vi "Configure Measurement.vi"(6 "Manual Range (1.00)":dbl=1.0 format="%_3f", 7 "Manual Resolution (5.5 Digits)":dbl(ring)=5.5 items=["4.5"=4.5, "5.5"=5.5, "6.5"=6.5], 8 "error in (no error)":errorcluster, 9 "Enable Auto Range (T: Enable)":bool=TRUE, 10 "Function (0: DC Voltage)":u16(ring) items=["DC Voltage", "AC Voltage", "2 - Wire Resistance", "4 - Wire Resistance", "DC Current", "AC Current", "Frequency", "Period", "Continuity", "Diode Checking", "VDC:VDC Ratio", "Temperature", "Capacitance"], 11 "VISA resource name":refnum<visa-resource-name>) -> (0 "error out":errorcluster, 3 "VISA resource name out":refnum<visa-resource-name>)   [LabVIEW 2013, in "Agilent 34401.lvlib"]
doc: "Configures the measurement type, resolution, and range on the instrument.\n\n<B>Note:</B>\n\nThis VI must be called before other configuration VIs."
uses:
  <instrlib>/Agilent 34401/Agilent 34401.lvlib
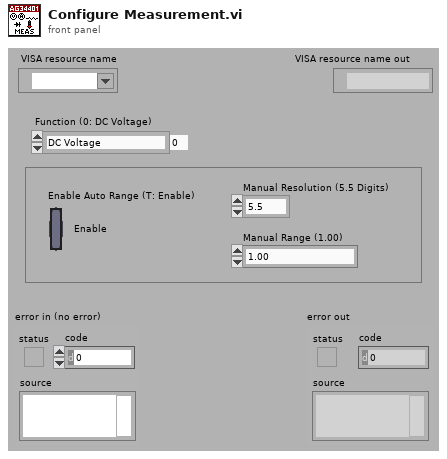
[diagram p1: front panel]
types:
  T1 = typedef "Agilent 34401.lvlib/Extended User Data.ctl" = cluster{"Trigger Source":u16, "Math Storage":u16, "Agilent Model":i32}
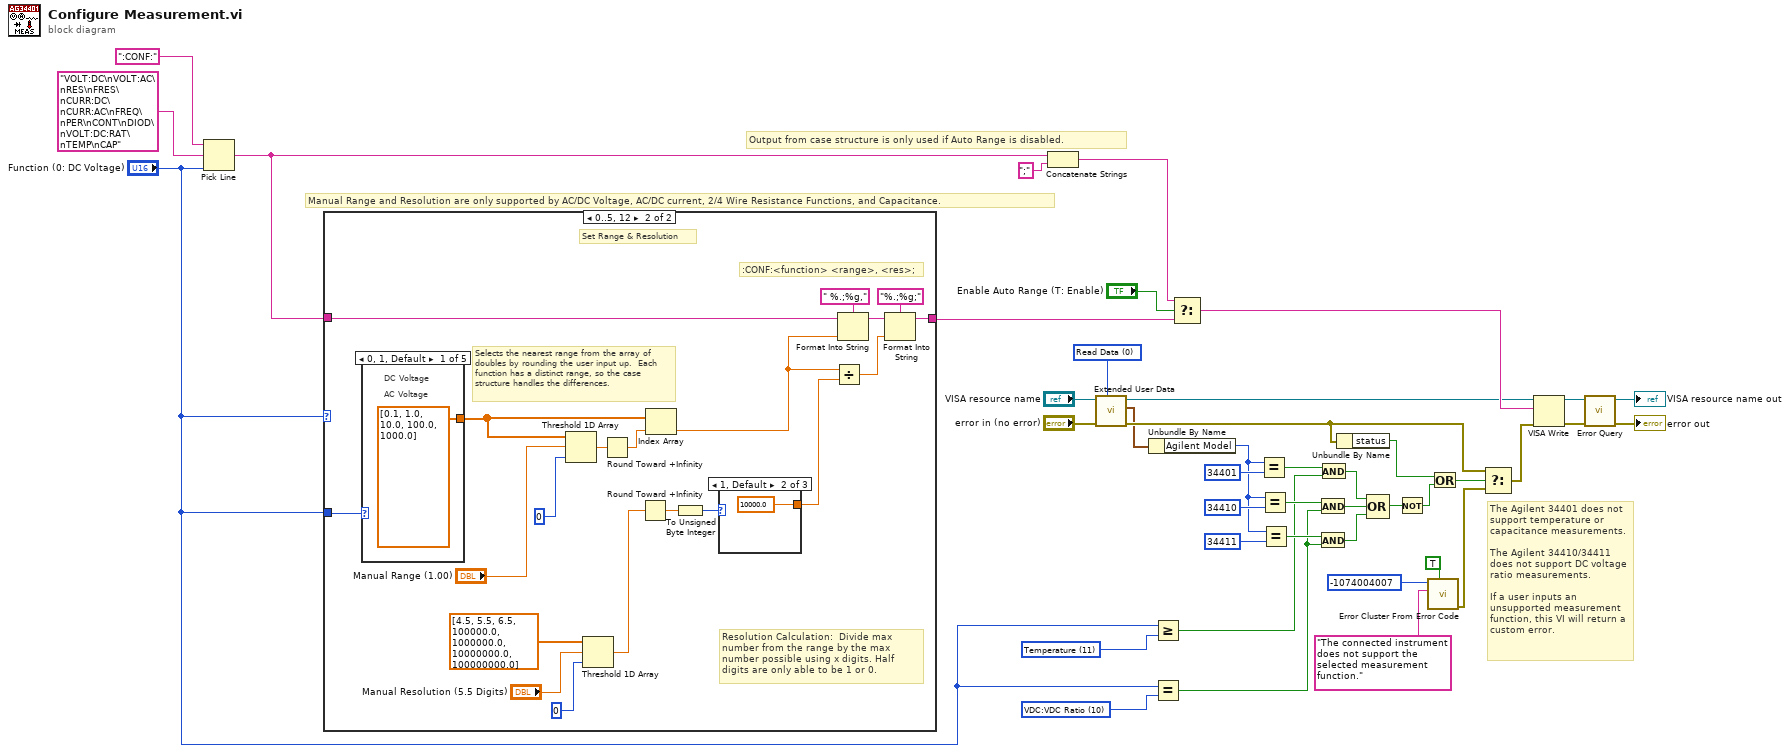
[diagram p0: block diagram]
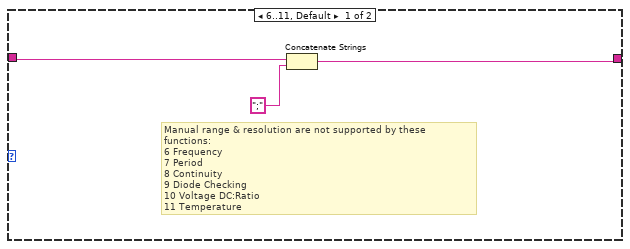
[diagram p2: hidden frame]
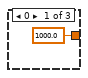
[diagram p3: hidden frame]
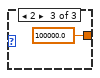
[diagram p4: hidden frame]
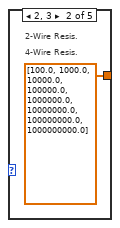
[diagram p5: hidden frame]
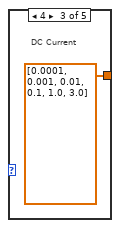
[diagram p6: hidden frame]
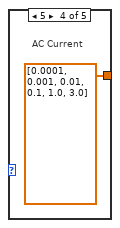
[diagram p7: hidden frame]
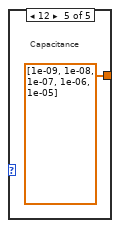
[diagram p8: hidden frame]
diagram:
  w4 = u16 10 items=["DC Voltage", "AC Voltage", "2 - Wire Resistance", "4 - Wire Resistance", "DC Current", "AC Current", "Frequency", "Period", "Continuity", "Diode Checking", "VDC:VDC Ratio", "Temperature", "Capacitance"] ("Function (0: DC Voltage)")
  w3 = u16 11 items=["DC Voltage", "AC Voltage", "2 - Wire Resistance", "4 - Wire Resistance", "DC Current", "AC Current", "Frequency", "Period", "Continuity", "Diode Checking", "VDC:VDC Ratio", "Temperature", "Capacitance"] ("Function (0: DC Voltage)")
  w6 = u16 0 items=["Read Data", "Write Data", "Dispose of Data"] ("Action")
  # "The Agilent 34401 does not support temperature or capacitance measurements.\n\nThe Agilent 34410/34411 does not support DC voltage ratio measurements.\n\nIf a user inputs an unsupported measurement function, this VI will return a custom error."
  # "Manual Range and Resolution are only supported by AC/DC Voltage, AC/DC current, 2/4 Wire Resistance Functions, and Capacitance."
  # "Output from case structure is only used if Auto Range is disabled."
  n1 = Pick Line(string ("")=":CONF:", multi-line string="VOLT:DC\nVOLT:AC\nRES\nFRES\nCURR:DC\nCURR:AC\nFREQ\nPER\nCONT\nDIOD\nVOLT:DC:RAT\nTEMP\nCAP", line index="Function (0: DC Voltage)") -> (output string=w31:string)
  n2 = case shown="0..5, 12" "Function (0: DC Voltage)" {
    tunnel: w31 -> [w45 w46]
    tunnel: "Function (0: DC Voltage)" -> [_ w56]
    tunnel: [w43 w54] -> w36
    frame 6..11, Default {
      # "Manual range & resolution are not supported by these functions:\n6 Frequency\n7 Period\n8 Continuity\n9 Diode Checking\n10 Voltage DC:Ratio\n11 Temperature"
      n3 = Concatenate Strings(w45, ";" ("Auto Range")) -> (w43:string)
    }
    frame 0..5, 12 {
      # "Set Range & Resolution"
      # ":CONF:<function> <range>, <res>;"
      # "Resolution Calculation:  Divide max number from the range by the max number possible using x digits. Half digits are only able to be 1 or 0."
      # "Selects the nearest range from the array of doubles by rounding the user input up.  Each function has a distinct range, so the case structure handles the differences."
      n4 = case shown="0, 1, Default" w56 {
        tunnel: [dbl[] [0.1, 1.0, 10.0, 100.0, 1000.0] ("Array Constant") dbl[] [100.0, 1000.0, 10000.0, 100000.0, 1000000.0, 10000000.0, 100000000.0, 1000000000.0] ("Array Constant") dbl[] [0.0001, 0.001, 0.01, 0.1, 1.0, 3.0] ("Array Constant") dbl[] [0.0001, 0.001, 0.01, 0.1, 1.0, 3.0] ("Array Constant") dbl[] [1e-09, 1e-08, 1e-07, 1e-06, 1e-05] ("Array Constant")] -> w57
        frame 0, 1, Default {
          # "AC Voltage"
          # "DC Voltage"
        }
        frame 2, 3 {
          # "4-Wire Resis."
          # "2-Wire Resis."
        }
        frame 4 {
          # "DC Current"
        }
        frame 5 {
          # "AC Current"
        }
        frame 12 {
          # "Capacitance"
        }
      }
      n5 = Threshold 1D Array(1:0 ("start index (0)"), 2:"Manual Range (1.00)", 3:w57) -> (0:w59:dbl)
      n6 = Threshold 1D Array(1:0 ("start index (0)"), 2:"Manual Resolution (5.5 Digits)", 3:dbl[] [4.5, 5.5, 6.5, 100000.0, 1000000.0, 10000000.0, 100000000.0] ("Array Constant")) -> (0:w51:dbl)
      n7 = Round Toward +Infinity ("Round To +Infinity")(x=w59) -> (ceil(x): smallest int >= x=w60:dbl)
      n8 = Round Toward +Infinity ("Round To +Infinity")(x=w51) -> (ceil(x): smallest int >= x=w49:dbl)
      n9 = Index Array(array=w57, index=w60) -> (element=w58:dbl)
      n10 = To Unsigned Byte Integer(number=w49) -> (unsigned 8bit integer=w50:u8)
      n11 = case shown="1, Default" w50 {
        tunnel: [1000.0 10000.0 100000.0] -> w53
        frame 0 {
        }
        frame 1, Default {
        }
        frame 2 {
        }
      }
      n12 = Divide(x=w58, y=w53) -> (x/y=w65:dbl)
      n13 = Format Into String(format string=" %.;%g,", initial string=w46, w58) -> (resulting string=w62:string)  [unwired: 1 in, 1 out]
      n14 = Format Into String(format string="%.;%g;", initial string=w62, w65) -> (resulting string=w54:string)  [unwired: 1 in, 1 out]
    }
  }
  n15 = Concatenate Strings(w31, ";" ("t")) -> (w33:string)
  n16 = call <instrlib>:"Extended User Data.vi"("Action"=w6, "Error In (no error)"="error in (no error)", "VISA resource name in"="VISA resource name") -> ("Error Out"=w9:errorcluster, "User Data Out"=w7:T1, "VISA resource name out"=w8:refnum<visa-resource-name>)  [unwired: 6 in]
  n17 = Unbundle By Name(w7) -> ("Agilent Model"=w5:i32)
  n18 = Greater Or Equal?(x="Function (0: DC Voltage)", y=w3) -> (x >= y?=w1:bool)
  n19 = Equal?(x="Function (0: DC Voltage)", y=w4) -> (x = y?=w23:bool)
  n20 = Select(t=w33, s="Enable Auto Range (T: Enable)", f=w36) -> (s? t:f=w34:string)
  n21 = Equal?(x=w5, y=34401) -> (x = y?=w21:bool)
  n22 = Equal?(x=w5, y=34410) -> (x = y?=w22:bool)
  n23 = Equal?(x=w5, y=34411) -> (x = y?=w24:bool)
  n24 = And(x=w22, y=w23) -> (x .and. y?=w20:bool)
  n25 = And(x=w24, y=w23) -> (x .and. y?=w18:bool)
  n26 = And(x=w21, y=w1) -> (x .and. y?=w19:bool)
  n27 = Unbundle By Name(w9) -> ("status"=w14:bool)
  n28 = Compound Arithmetic op=OR(w19, w20, w18) -> (w15:bool)
  n29 = Not(x=w15) -> (.not. x?=w13:bool)
  n30 = call <vilib>:"Error Cluster From Error Code.vi"("show call chain? (False)"=TRUE, "error message (\"\")"="The connected instrument does not support the selected measurement function." ("Source (VI Name)"), "error code (0)"=-1074004007 ("Code")) -> ("error out"=w17:errorcluster)  [unwired: 6 in]
  n31 = Or(x=w14, y=w13) -> (x .or. y?=w12:bool)
  n32 = Select(t=w9, s=w12, f=w17) -> (s? t:f=w16:errorcluster)
  n33 = VISA Write(VISA resource name=w8, write buffer=w34, error in (no error)=w16) -> (VISA resource name out=w40:refnum<visa-resource-name>, error out=w39:errorcluster)  [unwired: 1 out]
  n34 = call <instrlib>:"Error Query.vi"("error in (no error)"=w39, "VISA resource name"=w40) -> ("error out"=→"error out":errorcluster, "VISA resource name out"=→"VISA resource name out":refnum<visa-resource-name>)  [unwired: 6 in, 2 out]
